vi "Get UI Details.vi"() -> ()   [LabVIEW 2021, in "Single Tone_DAC.lvlib"]
uses:
  Single Tone_DAC.lvlib
  <vilib>/MeasurementLink/MeasurementLink Measurement Server/Helpers/TypeDefs/User Interface Information.ctl
  <vilib>/MeasurementLink/MeasurementLink Measurement Server/MeasurementLink Measurement Server.lvlib
panel:
  out "error out":errorcluster
  in  "error in":errorcluster
  out "user interface details":T1[](array[typedef])
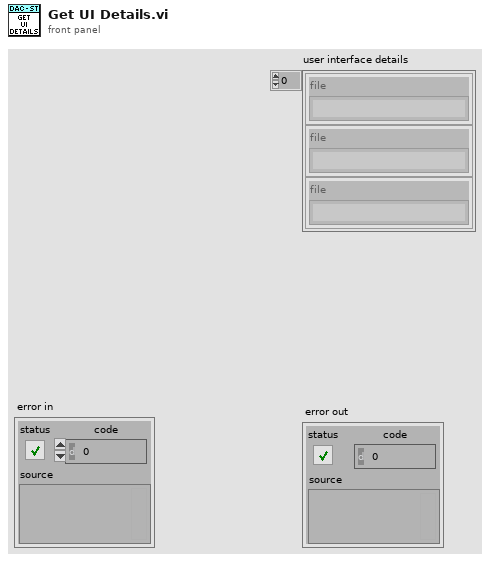
[diagram p1: front panel]
types:
  T1 = typedef "MeasurementLink Measurement Server.lvlib/User Interface Information.ctl" = cluster{"file":string}
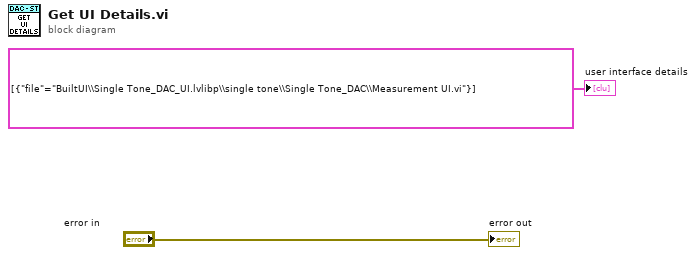
[diagram p0: block diagram]
diagram:
  "user interface details" <- T1[] [{"file"="BuiltUI\\Single Tone_DAC_UI.lvlibp\\single tone\\Single Tone_DAC\\Measurement UI.vi"}] ("appended array")
  "error out" <- "error in"
